vi "Set Control Properties.vi"(6 "VI Index":i32, 10 "Controls":string[][](array[string]), 11 "Item Data":refnum<class "Item.lvclass">[](array[class])) -> (3 "Item Data out":refnum<class "Item.lvclass">[](array[class]))   [LabVIEW 2020, in "VI Properties Editor.lvlib"]
doc: "Sets all new control properties of the VI identified by <B>VI Index</B>."
uses:
  VI Properties Editor.lvlib
  Classes/Item/Item.lvclass
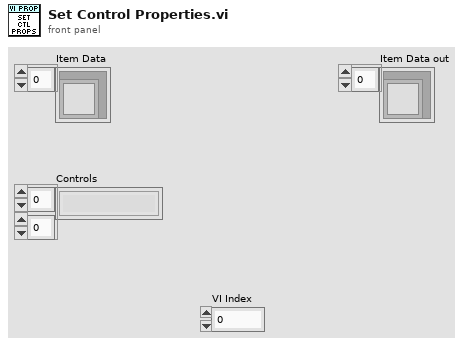
[diagram p1: front panel]
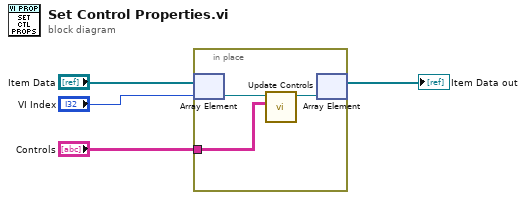
[diagram p0: block diagram]
diagram:
  n1 = in-place {
    in-place-border: "Controls" -> [w6]
    n2 = in-place-array #1("Item Data", "VI Index") -> (w7:refnum<class "Item.lvclass">)
    n3 = call-dynamic "Update Controls.vi"("Control Array"=w6, "Item in"=w7) -> ("Item out"=w5:refnum<class "Item.lvclass">)  [unwired: 8 in, 1 out]
    n4 = in-place-array #1(w5) -> (→"Item Data out":refnum<class "Item.lvclass">[])  [unwired: 1 out]
  }
